vi "Memory.Pointer.External.New Offset Pointer.vi"(7 "length (-1: rest)":i64=-1 format="%d bytes", 8 "error in (no error)":errorcluster, 9 "offset (0)":u64 format="%d bytes", 10 "offset pointer type":refnum<class "Memory.Pointer.External.lvclass">, 11 "base pointer in":refnum<class "Memory.Pointer.lvclass">) -> (0 "error out":errorcluster, 2 "offset pointer":refnum<class "Memory.Pointer.External.lvclass">, 3 "base pointer out":refnum<class "Memory.Pointer.lvclass">)   [LabVIEW 2016, in "Memory.lvlib" / "Memory.Pointer.External.lvclass"]
uses:
  Memory.Pointer.External.lvclass
  Pointer/Memory.Pointer.lvclass
  Pointer/Memory.Pointer.lvclass/Memory.Pointer.ctl
  Pointer/Memory.Pointer.Errors.vi
  Pointer/Memory.Pointer.Errors.Out of Bounds.vi
  Pointer/Memory.Pointer.Get Size.vi
  Pointer/Memory.Pointer.Errors.Null Pointer.vi
  Submodules/SEH/Source/VIs/Static Error Handling.Source Buffer.Write.String.vi
  Pointer/Memory.Pointer.Errors.Write Pointer Size.vi
  Pointer/Memory.Pointer.Errors.Create Error.vi
  Submodules/SEH/Source/VIs/Static Error Handling.Source Buffer.Write.Numeric.Scalar.Base10.vi
  Submodules/SEH/Source/VIs/Static Error Handling.Source Buffer.Write.Numeric.Scalar.Base10 (U64).vi
  Submodules/SEH/Source/VIs/Static Error Handling.Error Cluster Constant.vi
  Submodules/SEH/Source/VIs/Static Error Handling.Error Cluster Constant (256B).vi
  Submodules/SEH/Source/VIs/Static Error Handling.Parameters.Status.Set.vi
  Submodules/SEH/Source/VIs/Static Error Handling.Parameters.Code.Set.vi
  Submodules/SEH/Source/VIs/Static Error Handling.Parameters.VI Source.Set.vi
  Constants/Memory.Constants.vi
  Constants/Memory.Constants.Library Name.vi
  Pointer/Memory.Pointer.Errors.Get Info.vi
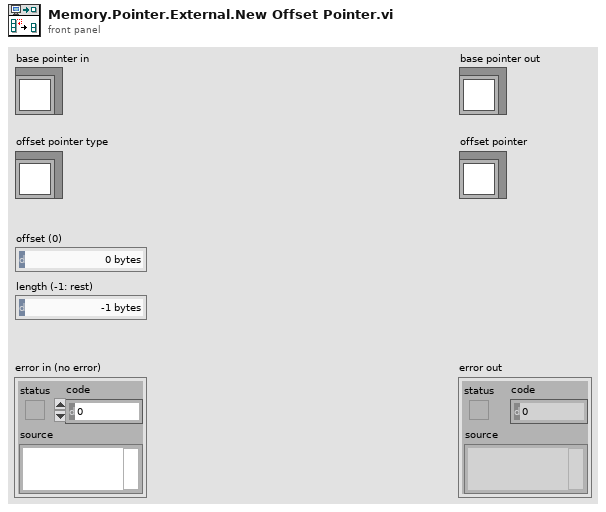
[diagram p1: front panel]
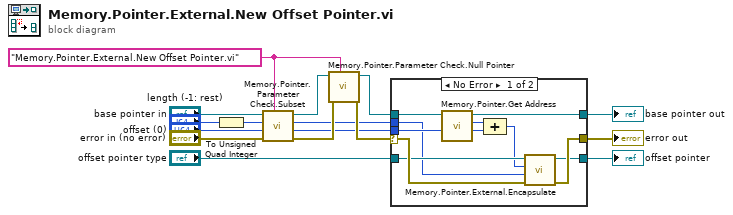
[diagram p0: block diagram]
diagram:
  w2 = "Memory.Pointer.External.New Offset Pointer.vi" ("source vi name")
  n1 = To Unsigned Quad Integer(1:"length (-1: rest)") -> (0:w12:u64)
  n2 = call "Memory.Pointer.Parameter Check.Subset.vi"("source vi name"=w2, "error in (no error)"="error in (no error)", "offset (0)"="offset (0)", "length"=w12, "Pointer in"="base pointer in") -> ("error out"=w16:errorcluster, "offset out"=w5:u64, "length"=w6:u64, "Pointer out"=w4:refnum<class "Memory.Pointer.lvclass">)  [unwired: 3 in]
  n3 = call "Memory.Pointer.Parameter Check.Null Pointer.vi"("source vi name"=w2, "error in (no error)"=w16, "Pointer in"=w4) -> ("error out"=w15:errorcluster, "Pointer out"=w3:refnum<class "Memory.Pointer.lvclass">)  [unwired: 7 in]
  n4 = case shown="No Error" w15 {
    selector: w15 -> [w26 w27]
    tunnel: "offset pointer type" -> [w25 w28]
    tunnel: [w23 w28] -> w8
    tunnel: w3 -> [w22 w29]
    tunnel: [w21 w29] -> w7
    tunnel: w6 -> [w17 _]
    tunnel: w5 -> [w20 _]
    tunnel: [w24 w27] -> w1
    frame No Error {
      n5 = call "Memory.Pointer.Get Address.vi"("Pointer in"=w22) -> ("address"=w19:u64, "Pointer out"=w21:refnum<class "Memory.Pointer.lvclass">)  [unwired: 9 in]
      n6 = Compound Arithmetic op=ADD(w19, w20) -> (w18:u64)
      n7 = call "Memory.Pointer.External.Encapsulate.vi"("error in (no error)"=w26, "size"=w17, "address"=w18, "external pointer type"=w25) -> ("error out"=w24:errorcluster, "external pointer out"=w23:refnum<class "Memory.Pointer.External.lvclass">)  [unwired: 6 in]
    }
    frame Error {
    }
  }
  "error out" <- w1
  "offset pointer" <- w8
  "base pointer out" <- w7
